vi "CAPTH-Release IPC.vi"(7 "IPC":T1) -> ()   [LabVIEW 2020]
uses:
  Typedefs/CAPTH-IPC.ctl
  Typedefs/CAPTH-Start Data.ctl
  Typedefs/CAPTH-Parameters.ctl
  Typedefs/CAPTH-Stimulus.ctl
  Typedefs/CAPTH-Response.ctl
  Typedefs/CAPTH-Analysis Message.ctl
  Typedefs/CAPTH-Analysis Action.ctl
  Typedefs/CAPTH-StimCon.ctl
  Typedefs/CAPTH-Analysis Data Properties.ctl
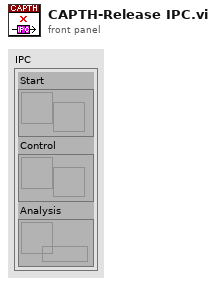
[diagram p1: front panel]
types:
  T1 = typedef "CAPTH-IPC.ctl" = cluster{"Start":refnum<notifier>, "Control":refnum<notifier>, "Analysis":refnum<queue>}
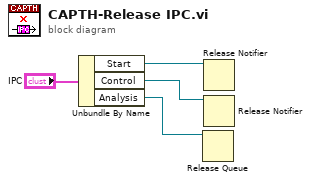
[diagram p0: block diagram]
diagram:
  n1 = Unbundle By Name("IPC") -> ("Start"=w3:refnum<notifier>, "Control"=w2:refnum<notifier>, "Analysis"=w1:refnum<queue>)
  n2 = Release Queue(queue=w1) -> ()  [unwired: 2 in, 3 out]
  n3 = Release Notifier(notifier=w3) -> ()  [unwired: 2 in, 3 out]
  n4 = Release Notifier(notifier=w2) -> ()  [unwired: 2 in, 3 out]
